vi "GetSfxDLData.vi"(5 "Resp Timeout (ms)":i32 min=0, 6 "Rx Timeout (ms)":u32=1, 7 "Enum":T1, 8 "Error In":errorcluster, 9 "Freq Offset (Hz)":i32=1, 10 "Rx Freq (Hz)":u32=1, 11 "FPGA Reference":refnum<k20>) -> (0 "Error Out":errorcluster, 1 "Rx Payload (Hex)":string, 2 "Get DL OK":bool, 3 "Received Text":string, 4 "RSSI (dBm)":i16)   [LabVIEW 2018]
uses:
  Resources_Test/UART/ControlTestSlot.ctl
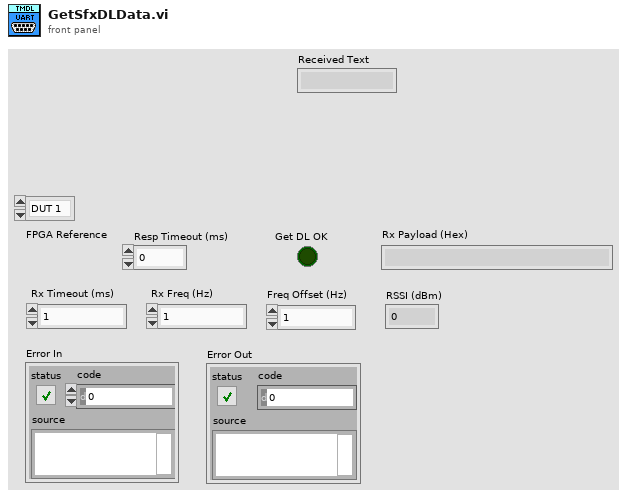
[diagram p1: front panel]
types:
  T1 = typedef "ControlTestSlot.ctl" = enum16{"DUT 1", "DUT 2"}
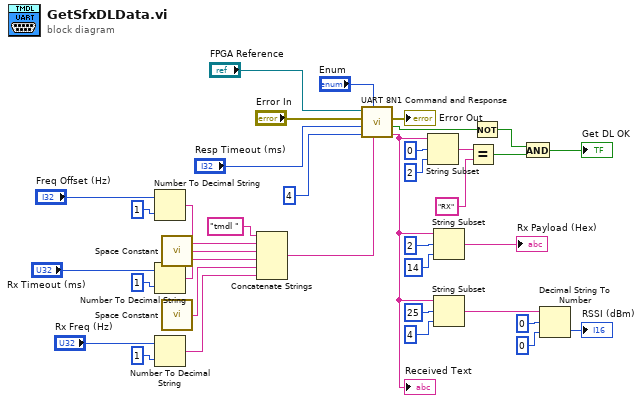
[diagram p0: block diagram]
diagram:
  n1 = Number To Decimal String(number="Freq Offset (Hz)", width (-)=i16 1) -> (decimal integer string=w29:string)
  n2 = Number To Decimal String(number="Rx Timeout (ms)", width (-)=i16 1) -> (decimal integer string=w27:string)
  n3 = Number To Decimal String(number="Rx Freq (Hz)", width (-)=i16 1) -> (decimal integer string=w24:string)
  n4 = call <vilib>:"Space Constant.vi"() -> ("String"=w28:string)
  n5 = call <vilib>:"Space Constant.vi"() -> ("String"=w26:string)
  n6 = Concatenate Strings("tmdl " ("Text to Send"), w29, w28, w27, w26, w24) -> (w4:string)
  n7 = call "UART 8N1 Command and Response.vi"("Text to Send"=w4, "Active Dut"="Enum", "Response Size (char)"=u32 4, "Response Timeout (ms)"="Resp Timeout (ms)", "Error In"="Error In", "FPGA VI Reference In"="FPGA Reference") -> ("Received Text"=w1:string, "Timeout Flag"=w2:bool, "Error Out"=→"Error Out":errorcluster)  [unwired: 1 in, 2 out]
  "Received Text" <- w1
  n8 = String Subset(string=w1, offset (0)=0, length (rest)=2 ("length (rest)")) -> (substring=w21:string)
  n9 = String Subset(string=w1, offset (0)=2, length (rest)=14 ("length (rest)")) -> (substring=→"Rx Payload (Hex)":string)
  n10 = String Subset(string=w1, offset (0)=25, length (rest)=4 ("length (rest)")) -> (substring=w15:string)
  n11 = Equal?(x=w21, y="RX") -> (x = y?=w35:bool)
  n12 = Not(x=w2) -> (.not. x?=w37:bool)
  n13 = And(x=w37, y=w35) -> (x .and. y?=→"Get DL OK":bool)
  n14 = Decimal String To Number(string=w15, offset=0, default (0L)=i16 0 ("default (0 I32)")) -> (number=→"RSSI (dBm)":i16)  [unwired: 1 out]
